vi "Go To Starting.vi"(8 "error in (no error)":errorcluster) -> (0 "error out":errorcluster)   [LabVIEW 2013, in "Command State.lvclass"]
uses:
  Command State.lvclass
  <vilib>/ni/Actors/State Actor/State Actor/State Actor.lvclass
  Starting/Starting.lvclass
panel:
  out "State out":refnum<class "State Actor.lvclass">
  in  "Command.lvlib:CommandStates.lvclass":refnum<class "Command State.lvclass">
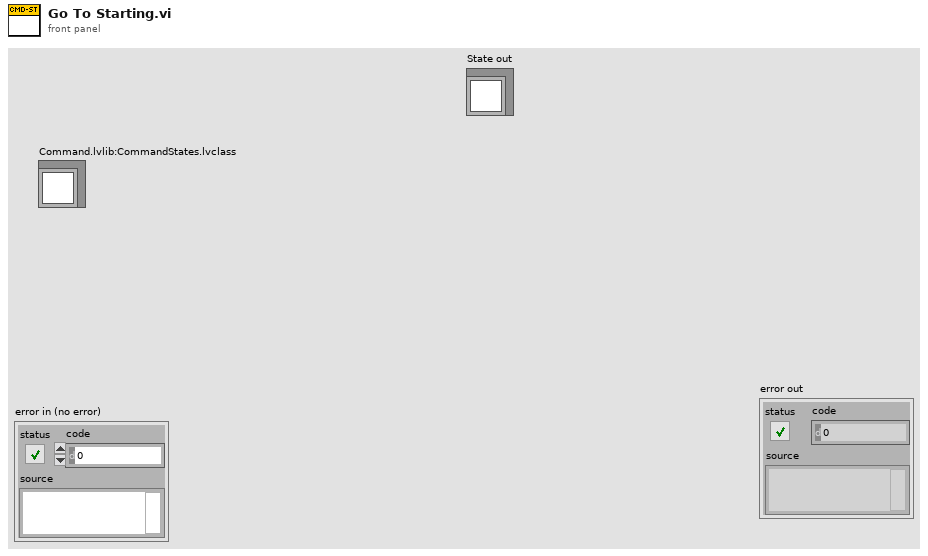
[diagram p1: front panel]
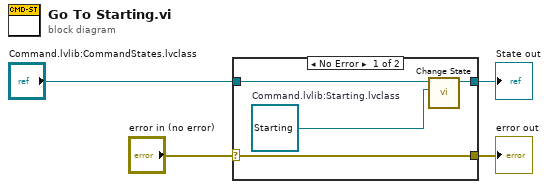
[diagram p0: block diagram]
diagram:
  n1 = case shown="No Error" "error in (no error)" {
    selector: "error in (no error)" -> [w8 w10]
    tunnel: [w8 w10] -> w3
    tunnel: "Command.lvlib:CommandStates.lvclass" -> [w7 w9]
    tunnel: [w6 w9] -> w1
    frame No Error {
      w5 = refnum<class "Starting.lvclass"> refnum  # Command.lvlib:Starting.lvclass
      n2 = call <vilib>:"Change State.vi"("New State in"=w5, "State in"=w7) -> ("State out"=w6:refnum<class "State Actor.lvclass">)  [unwired: 8 in, 1 out]
    }
    frame Error {
    }
  }
  "error out" <- w3
  "State out" <- w1
